vi "cRIO_FPGA_COMMUNICATION Behandle FPGA Lesen und Auswerten Daten.vi"(8 "Band- & Stationsdaten":u16[](array[numeric]), 10 "Station Index":T3, 11 "FGV Band/Station Commands":T2=enum."Schreibe") -> (3 "Band/Station Lese Daten":T1)   [LabVIEW 2013, in "cRIO_FPGA_COMMUNICATION.lvlib"]
uses:
  cRIO_FPGA_COMMUNICATION.lvlib
  TYPES/TYPE Station Index.ctl
  TYPES/TYPE Band und Stations Lese Kommandos.ctl
  TYPES/TYPE Band Lese Daten.ctl
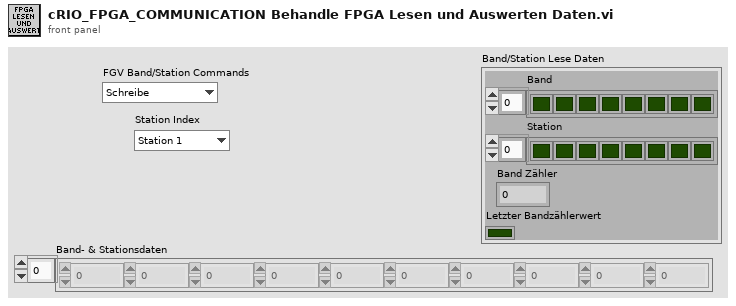
[diagram p1: front panel]
types:
  T1 = typedef "cRIO_FPGA_COMMUNICATION.lvlib/TYPE Band Lese Daten.ctl" = cluster{"Band":bool[], "Station":bool[], "Band Zähler":i32, "Letzter Bandzählerwert":bool}
  T2 = typedef "TYPE Band und Stations Lese Kommandos.ctl" = enum16{"Init", "Lese", "Schreibe"}
  T3 = typedef "cRIO_FPGA_COMMUNICATION.lvlib/TYPE Station Index.ctl" = enum16{"Station 1", "Station 2", "Station 3", "Station 4", "Station 5", "Station 6", "Station 7", "Station 8", "Station 9", "Station 10", "Station 11", "Station 12", "Station 13", "Station 14", "Station 15", "Station 16", "Station 17", "Station 18", "Station 19", "Station 20"}
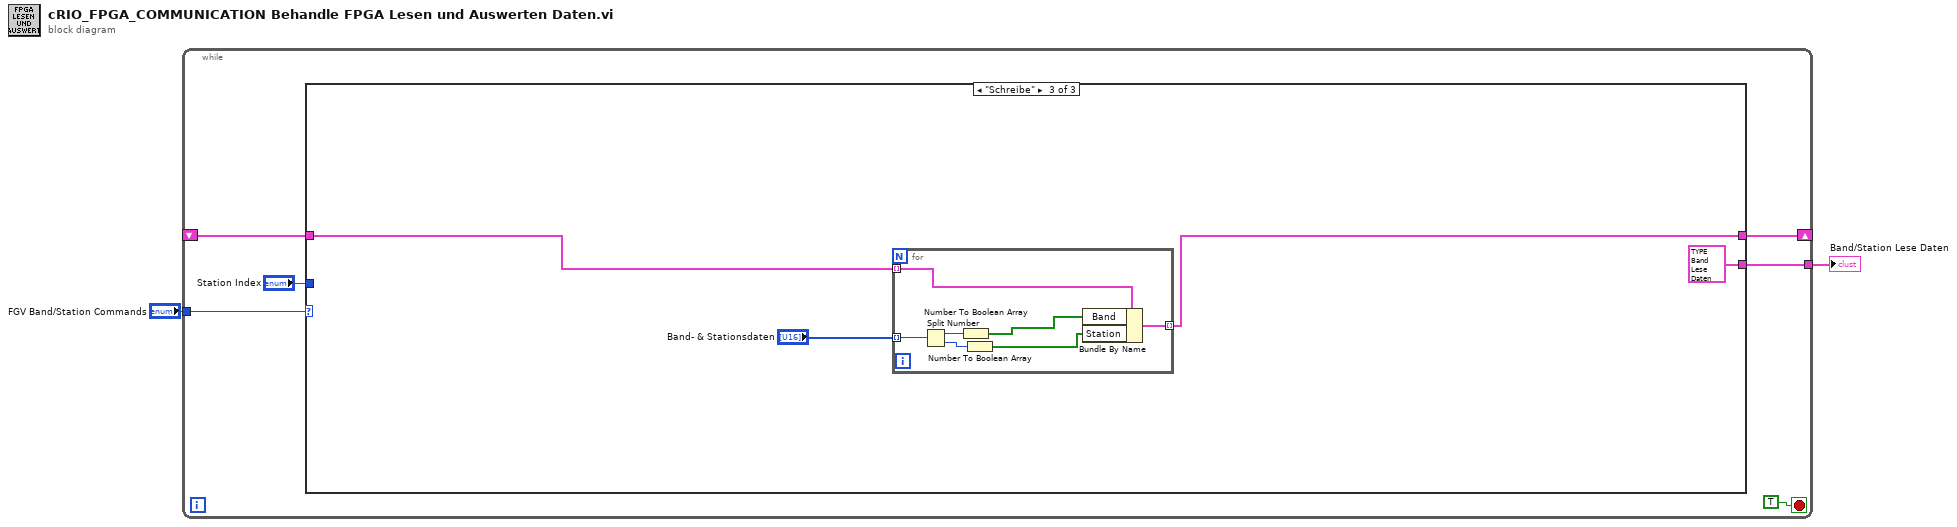
[diagram p0: block diagram]
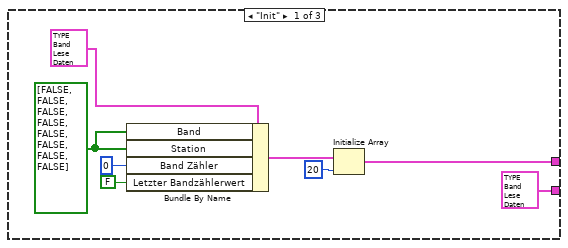
[diagram p2: hidden frame]
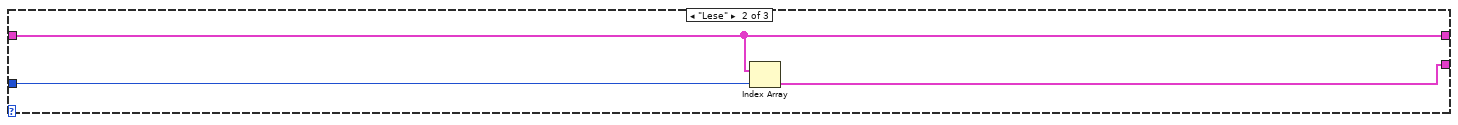
[diagram p3: hidden frame]
diagram:
  n1 = while {
    tunnel: "FGV Band/Station Commands" -> [w7]
    shift-right: [w6] -> _
    shift-left: _ -> [w5]
    tunnel: [w4] -> w1
    stop <- TRUE stop-if-true
    n2 = case shown="\"Schreibe\"" w7 {
      tunnel: [w13 w19 w22] -> w6
      tunnel: w5 -> [_ w19 w23]
      tunnel: [T1 {"Band"=[FALSE, FALSE, FALSE, FALSE, FALSE, FALSE, FALSE, FALSE], "Station"=[FALSE, FALSE, FALSE, FALSE, FALSE, FALSE, FALSE, FALSE], "Band Zähler"=0, "Letzter Bandzählerwert"=FALSE} ("Band Lese Daten") w18 T1 {"Band"=[FALSE, FALSE, FALSE, FALSE, FALSE, FALSE, FALSE, FALSE], "Station"=[FALSE, FALSE, FALSE, FALSE, FALSE, FALSE, FALSE, FALSE], "Band Zähler"=0, "Letzter Bandzählerwert"=FALSE} ("Band Lese Daten")] -> w4
      tunnel: "Station Index" -> [_ w17 _]
      frame "Init" {
        w15 = bool[] [FALSE, FALSE, FALSE, FALSE, FALSE, FALSE, FALSE, FALSE] ("Band")
        n3 = Bundle By Name(cluster=T1 {"Band"=[FALSE, FALSE, FALSE, FALSE, FALSE, FALSE, FALSE, FALSE], "Station"=[FALSE, FALSE, FALSE, FALSE, FALSE, FALSE, FALSE, FALSE], "Band Zähler"=0, "Letzter Bandzählerwert"=FALSE} ("Band Lese Daten"), "Band"=w15, "Station"=w15, "Band Zähler"=0, "Letzter Bandzählerwert"=FALSE) -> (w14:T1)
        n4 = Initialize Array(w14, 20 ("Dimension")) -> (w13:T1[])
      }
      frame "Lese" {
        n5 = Index Array(array=w19, index=w17) -> (element=w18:T1)
      }
      frame "Schreibe" {
        n6 = for {
          tunnel: w23 -> [w28] mode=indexing
          tunnel: [w25] -> w22 mode=indexing
          tunnel: "Band- & Stationsdaten" -> [w24] mode=indexing
          n7 = Split Number(x=w24) -> (hi(x)=w30:u8, lo(x)=w29:u8)
          n8 = Number To Boolean Array(number=w30) -> (Boolean array=w27:bool[])
          n9 = Number To Boolean Array(number=w29) -> (Boolean array=w26:bool[])
          n10 = Bundle By Name(cluster=w28, "Band"=w27, "Station"=w26) -> (w25:T1)
        }
      }
    }
  }
  "Band/Station Lese Daten" <- w1
